vi "VA CoAP - Server - Proccess Message.vi"(0 "Conn IN":refnum<k16>, 5 "JSON Value in":refnum<class "JSON Value.lvclass">, 11 "error in (no error)":errorcluster) -> (4 "connection ID out":refnum<k16>, 6 "JSON Value out":refnum<class "JSON Value.lvclass">, 15 "error out":errorcluster)   [LabVIEW 2020]
uses:
  <vilib>/addons/JSON API/JSON Value/JSON Value.lvclass
  data types/VA CoAP - Message - Type.ctl
  <vilib>/addons/Tools/Unicode/UTF8 Tools.lvlib
panel:
  in  "CoAP Message 3":u8[](array[numeric]) format="%x"
  out "CoAP Message 2":u8[](array[numeric]) format="%x"
  out "CoAP Message":string
  out "Process?":bool
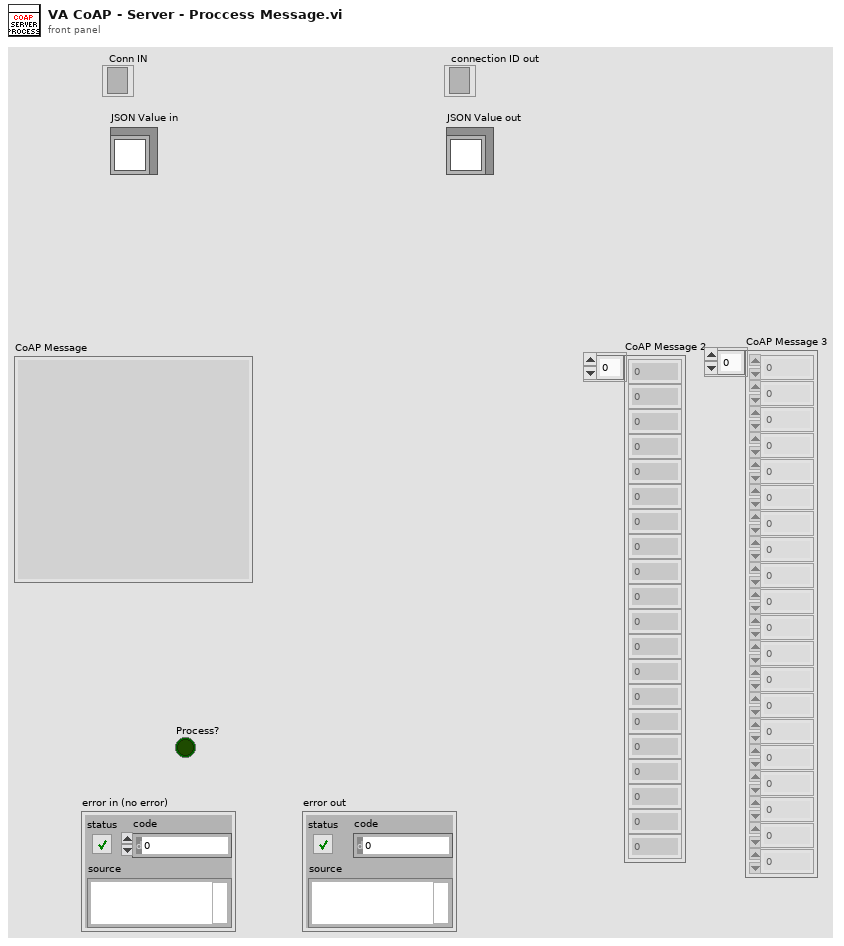
[diagram p1: front panel]
types:
  T1 = typedef "VA CoAP - Message.ctl" = cluster{"Type":T2, "Code":string, "Message ID":u16, "Token":string, "Options":T3, "Payload":string}
  T2 = typedef "VA CoAP - Message - Type.ctl" = u8
  T3 = typedef "VA CoAP - Message - Options.ctl" = cluster{"11: Uri-Path":T4}
  T4 = typedef "VA CoAP - Message - Options - 11 Uri-Path.ctl" = string[]
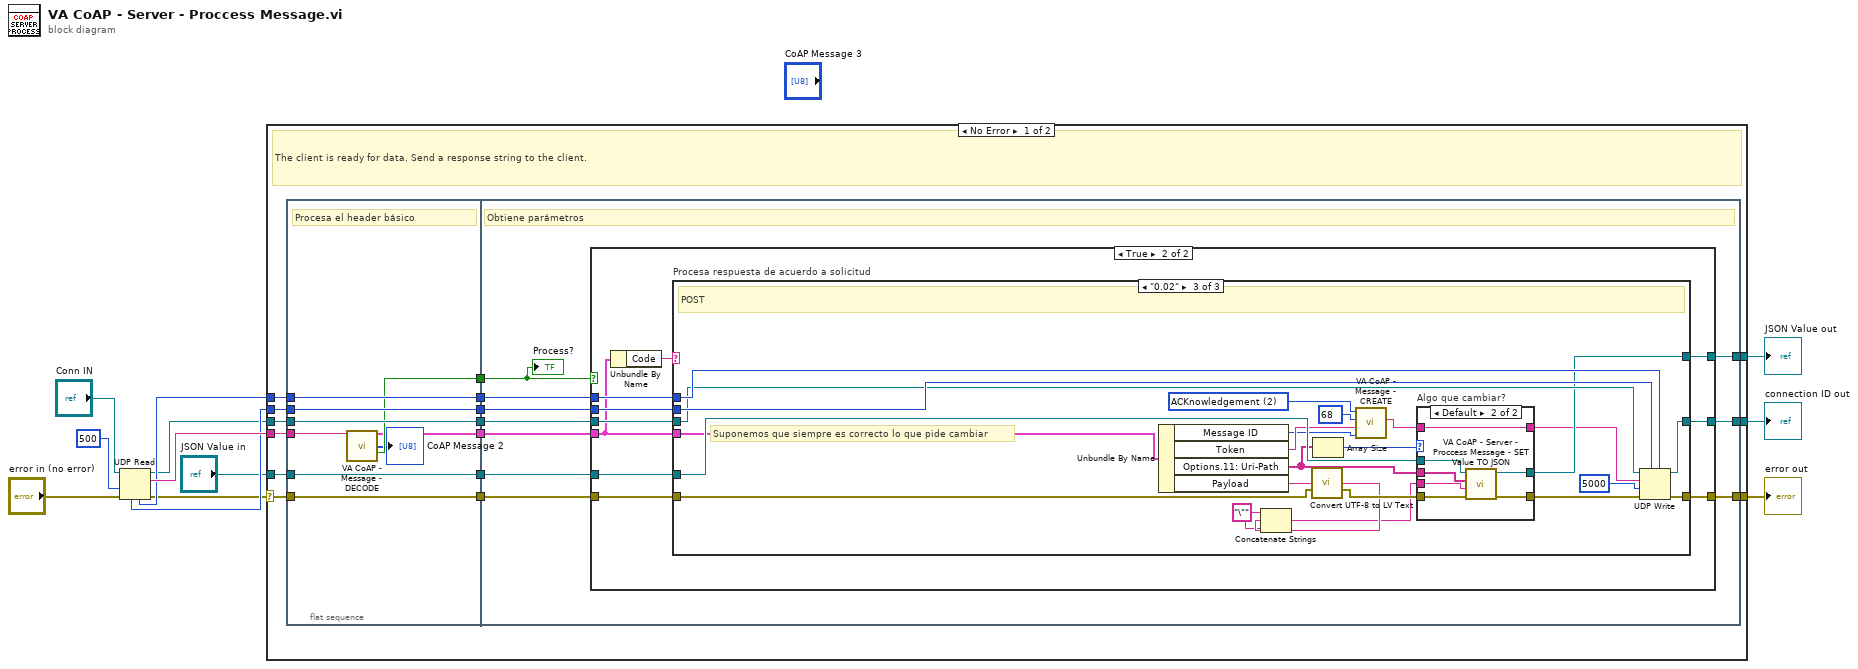
[diagram p0: block diagram]
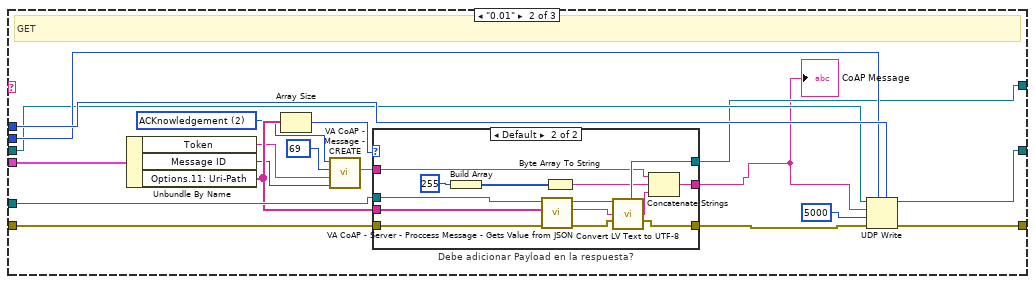
[diagram p4: hidden frame]
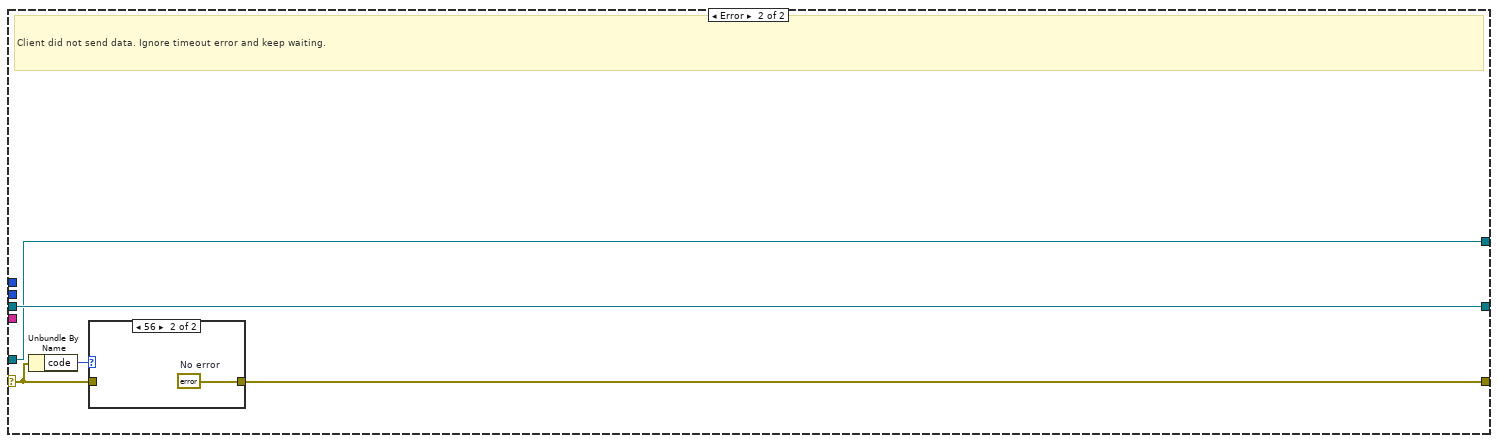
[diagram p7: hidden frame]
diagram:
  n1 = UDP Read(connection ID="Conn IN", timeout ms (25000)=500, 8:"error in (no error)") -> (data out=w12:string, error out=w1:errorcluster, 3:w5:refnum<k16>, 4:w8:u16, 6:w11:u32)  [unwired: 1 in]
  n2 = case shown="No Error" w1 {
    selector: w1 -> [w20 w136]
    tunnel: w5 -> [w16 w137]
    tunnel: [w26 w134] -> w9
    tunnel: [w27 w137] -> w6
    tunnel: w11 -> [w18 _]
    tunnel: w8 -> [w23 _]
    tunnel: w12 -> [w28 _]
    tunnel: "JSON Value in" -> [w21 w133]
    tunnel: [w25 w133] -> w2
    frame No Error {
      # "The client is ready for data. Send a response string to the client."
      n3 = flat-sequence {
        tunnel: w28 -> [w34]
        tunnel: [w37] -> w24
        tunnel: w23 -> [w37]
        tunnel: [w33] -> w22
        tunnel: w21 -> [w33]
        tunnel: w20 -> [w32]
        tunnel: [w36] -> w19
        tunnel: w18 -> [w36]
        tunnel: [w35] -> w17
        tunnel: w16 -> [w35]
        tunnel: [w32] -> w15
        tunnel: [w30] -> w14
        tunnel: [w31] -> w13
        tunnel: [w47] -> w26
        tunnel: [w46] -> w27
        tunnel: [w45] -> w25
        tunnel: w24 -> [w44]
        tunnel: w22 -> [w43]
        tunnel: w19 -> [w42]
        tunnel: w17 -> [w41]
        tunnel: w15 -> [w40]
        tunnel: w14 -> [w39]
        tunnel: w13 -> [w38]
        frame #0 {
          # "Procesa el header básico"
          n4 = call "VA CoAP - Message - DECODE.vi"("CoAP Message"=w34) -> ("CoAP Message Decoded"=w30:T1, "CoAP Message"=→"CoAP Message 2":u8[], "Valid?"=w31:bool)  [unwired: 11 in, 1 out]
        }
        frame #1 {
          # "Obtiene parámetros"
          n5 = case shown="True" w38 {
            tunnel: w44 -> [_ w60]
            tunnel: w42 -> [_ w59]
            tunnel: w41 -> [w50 w58]
            tunnel: [w48 w57] -> w47
            tunnel: [w50 w56] -> w46
            tunnel: w43 -> [w49 w54]
            tunnel: [w49 w55] -> w45
            tunnel: w40 -> [w48 w53]
            tunnel: w39 -> [_ w52]
            frame False {
            }
            frame True {
              n6 = Unbundle By Name(w52) -> ("Code"=w51:string)
              n7 = case "Procesa respuesta de acuerdo a solicitud" shown="\"0.02\"" w51 {
                tunnel: w60 -> [_ w82 w122]
                tunnel: w59 -> [_ w81 w121]
                tunnel: w58 -> [w61 w80 w120]
                tunnel: [w62 w79 w119] -> w57
                tunnel: [w61 w78 w118] -> w56
                tunnel: [w63 w77 w117] -> w55
                tunnel: w54 -> [w63 w76 w116]
                tunnel: w53 -> [w62 w75 w104]
                tunnel: w52 -> [_ w70 w107]
                frame Default {
                }
                frame "0.01" {
                  w69 = T2 2 items=["CONfimable", "NON-confirmable", "ACKnowledgement", "ReSeT"] ("Type")
                  # "GET"
                  n8 = Unbundle By Name(w70) -> ("Token"=w67:string, "Message ID"=w66:u16, "Options.11: Uri-Path"=w71:T4)
                  n9 = Array Size(array=w71) -> (size(s)=w74:i32)
                  n10 = call "VA CoAP - Message - CREATE.vi"("Message ID"=w66, "Token"=w67, "Method Code"=u8 69, "Type"=w69) -> ("CoAP Message"=w72:string)  [unwired: 6 in]
                  n11 = case "Debe adicionar Payload en la respuesta?" shown="Default" w74 {
                    tunnel: w71 -> [_ w98]
                    tunnel: w76 -> [w85 w97]
                    tunnel: [w85 w96] -> w77
                    tunnel: w72 -> [w84 w95]
                    tunnel: [w84 w92] -> w64
                    tunnel: w75 -> [w83 w91]
                    tunnel: [w83 w86] -> w73
                    frame 0 {
                    }
                    frame Default {
                      n12 = Build Array(u8 255) -> (w93:u8[])
                      n13 = call "VA CoAP - Server - Proccess Message - Gets Value from JSON.vi"("error in (no error)"=w91, "Item name"=w98, "JSON Value in"=w97) -> ("error out"=w87:errorcluster, "Value"=w88:string, "JSON Value out"=w96:refnum<class "JSON Value.lvclass">)  [unwired: 6 in]
                      n14 = Byte Array To String(unsigned byte array=w93) -> (string=w90:string)
                      n15 = call <vilib>:"Convert LV Text to UTF-8.vi"("LV Text"=w88, "error in"=w87) -> ("UTF-8 Text"=w89:string, "error out"=w86:errorcluster)  [unwired: 12 in]
                      n16 = Concatenate Strings(w95, w90, w89) -> (w92:string)
                    }
                  }
                  "CoAP Message" <- w64
                  n17 = UDP Write(address=w81, port or service name=w82, connection ID=w80, data in=w64, 8:w73, 9:5000 ("timeout ms (25000)")) -> (error out=w79:errorcluster, 3:w78:refnum<k16>)
                }
                frame "0.02" {
                  w100 = "\"" ("string")
                  w111 = T2 2 items=["CONfimable", "NON-confirmable", "ACKnowledgement", "ReSeT"] ("Type")
                  # "Suponemos que siempre es correcto lo que pide cambiar"
                  # "POST"
                  n18 = Unbundle By Name(w107) -> ("Message ID"=w108:u16, "Token"=w109:string, "Options.11: Uri-Path"=w112:T4, "Payload"=w102:string)
                  n19 = call <vilib>:"Convert UTF-8 to LV Text.vi"("UTF-8 Text"=w102, "error in"=w104) -> ("LV Text"=w101:string, "error out"=w103:errorcluster)  [unwired: 12 in]
                  n20 = Concatenate Strings(w100, w101, w100) -> (w99:string)
                  n21 = Array Size(array=w112) -> (size(s)=w115:i32)
                  n22 = call "VA CoAP - Message - CREATE.vi"("Message ID"=w108, "Token"=w109, "Method Code"=u8 68, "Type"=w111) -> ("CoAP Message"=w113:string)  [unwired: 6 in]
                  n23 = case "Algo que cambiar?" shown="Default" w115 {
                    tunnel: w112 -> [_ w132]
                    tunnel: w116 -> [w125 w131]
                    tunnel: [w125 w130] -> w117
                    tunnel: w113 -> [w124 w126]
                    tunnel: [w124 w126] -> w105
                    tunnel: w103 -> [w123 w129]
                    tunnel: [w123 w128] -> w114
                    tunnel: w99 -> [_ w127]
                    frame 0 {
                    }
                    frame Default {
                      n24 = call "VA CoAP - Server - Proccess Message - SET Value TO JSON.vi"("error in (no error)"=w129, "New Value"=w127, "Item name"=w132, "JSON Value in"=w131) -> ("error out"=w128:errorcluster, "JSON Value out"=w130:refnum<class "JSON Value.lvclass">)  [unwired: 6 in]
                    }
                  }
                  n25 = UDP Write(address=w121, port or service name=w122, connection ID=w120, data in=w105, 8:w114, 9:5000 ("timeout ms (25000)")) -> (error out=w119:errorcluster, 3:w118:refnum<k16>)
                }
              }
            }
          }
          "Process?" <- w38
        }
      }
    }
    frame Error {
      # "Client did not send data. Ignore timeout error and keep waiting."
      n26 = Unbundle By Name(w136) -> ("code"=w135:i32)
      n27 = case shown="56" w135 {
        tunnel: w136 -> [w138 _]
        tunnel: [w138 w139] -> w134
        frame Default {
        }
        frame 56 {
          w139 = errorcluster {"status"=FALSE, "code"=0, "source"=""}  # No error
        }
      }
    }
  }
  "error out" <- w9
  "connection ID out" <- w6
  "JSON Value out" <- w2
